vi "ReadWriteFiles.vi"() -> ()   [LabVIEW 2019]
panel:
  in  "prompt (Open existing file)":string
  in  "file path (use dialog)":path
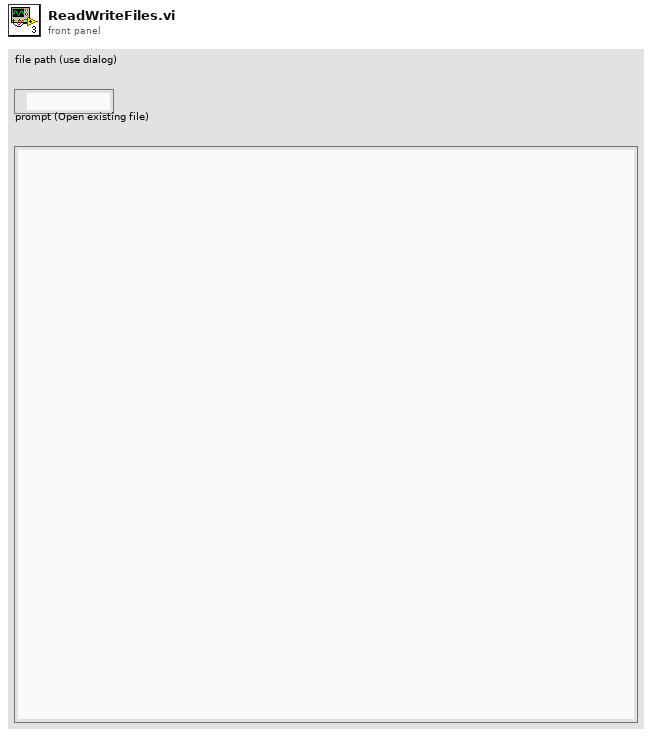
[diagram p1: front panel]
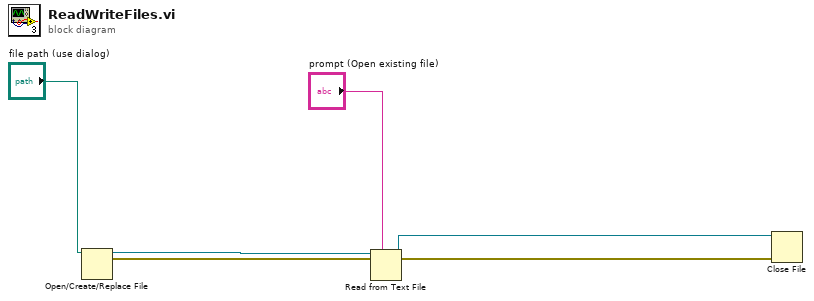
[diagram p0: block diagram]
diagram:
  n1 = Open/Create/Replace File(file path (use dialog)="file path (use dialog)") -> (refnum out=w5:refnum<file>, error out=w4:errorcluster)  [unwired: 5 in, 1 out]
  n2 = Read from Text File(prompt (Open existing file)="prompt (Open existing file)", file (use dialog)=w5) -> (refnum out=w3:refnum<file>)  [unwired: 2 in, 3 out]
  n3 = Close File(refnum=w3, error in=w4) -> ()  [unwired: 2 out]
